vi "Example--SMO.Example.vi"() -> ()   [LabVIEW 2013]
uses:
  SMO.Example/SMO.Example.lvclass
  SMO.UI.Example/SMO.UI.Example.lvclass
  SMO.Example/Typedefs/Configuration--Cluster.ctl
  SMO.UI.Example/SMO.UI.Example.lvclass/SMO.UI.Example.ctl
  SMO.UI/SMO.UI.lvclass
  SMO/SMO.lvclass
panel:
  in  "About":bool
  out "Data Changed":string
  out "error out":errorcluster
  in  "Stop":bool
  # "SMO Example Launcher"
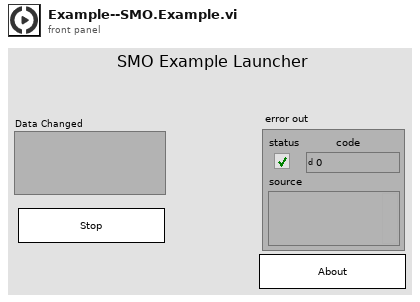
[diagram p1: front panel]
types:
  T1 = typedef "SMO.Example.lvclass/Configuration--Cluster.ctl" = cluster{"Suffix":string}
  T2 = cluster{"SMO out":refnum<class "SMO.Example.lvclass">}
  T3 = cluster{"SMO.Example Public Events":refnum<event-registration>, "SMO.UI Public Events":refnum<event-registration>}
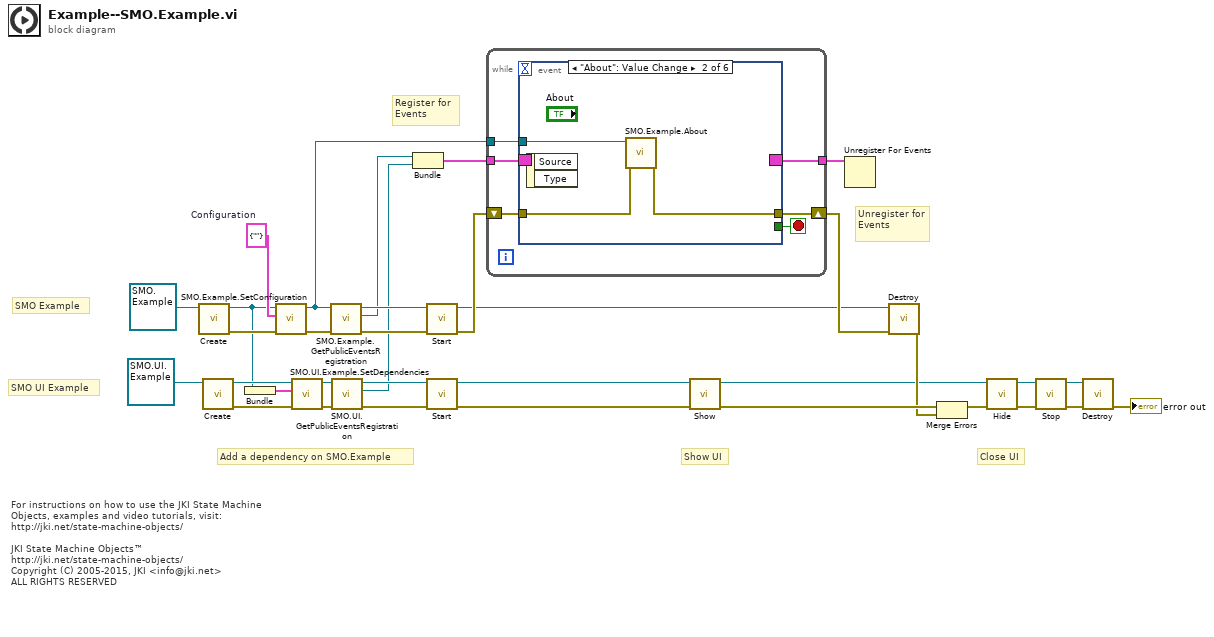
[diagram p0: block diagram]
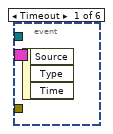
[diagram p2: hidden frame]
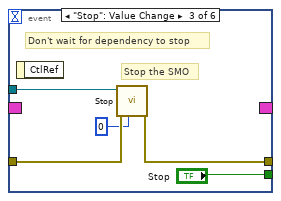
[diagram p3: hidden frame]
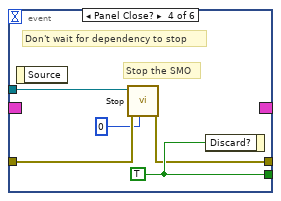
[diagram p4: hidden frame]
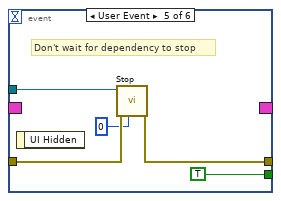
[diagram p5: hidden frame]
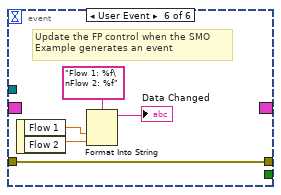
[diagram p6: hidden frame]
diagram:
  w23 = T1 {"Suffix"=""}  # Configuration
  # "Close UI"
  # "Show UI"
  # "SMO UI Example"
  # "SMO Example"
  # "For instructions on how to use the JKI State Machine Objects, examples and video tutorials, visit:\nhttp://jki.net/state-machine-objects/\n\nJKI State Machine Objects™\nhttp://jki.net/state-machine-objects/\nCopyright (C) 2005-2015, JKI <info@jki.net>\nALL RIGHTS RESERVED"
  # "Add a dependency on SMO.Example"
  # "Unregister for Events"
  # "Register for Events"
  n1 = call "Create.vi"("SMO"=refnum<class "SMO.Example.lvclass"> refnum ("SMO.Example.lvclass")) -> ("error out"=w22:errorcluster, "SMO out"=w6:refnum<class "SMO.Example.lvclass">)  [unwired: 8 in, 1 out]
  n2 = call "Create.vi"("SMO"=refnum<class "SMO.UI.Example.lvclass"> refnum ("SMO.UI.Example.lvclass")) -> ("error out"=w25:errorcluster, "SMO out"=w26:refnum<class "SMO.UI.Example.lvclass">)  [unwired: 8 in, 1 out]
  n3 = Bundle("SMO out"=w6) -> (w7:T2)  [unwired: 1 in]
  n4 = call "SMO.Example.SetConfiguration.vi"("error in (no error)"=w22, "Configuration"=w23, "SMO.Example"=w6) -> ("error out"=w18:errorcluster, "SMO.Example out"=w21:refnum<class "SMO.Example.lvclass">)  [unwired: 7 in]
  n5 = call "SMO.UI.Example.SetDependencies.vi"("error in (no error)"=w25, "Dependencies"=w7, "SMO UI.Template in"=w26) -> ("error out"=w17:errorcluster, "SMO UI.Template out"=w15:refnum<class "SMO.UI.Example.lvclass">)  [unwired: 7 in]
  n6 = call "SMO.Example.GetPublicEventsRegistration.vi"("error in (no error)"=w18, "SMO.Example"=w21) -> ("error out"=w19:errorcluster, "SMO.Example Public Events"=w12:refnum<event-registration>, "SMO.Example out"=w20:refnum<class "SMO.Example.lvclass">)  [unwired: 7 in]
  n7 = call "SMO.UI.GetPublicEventsRegistration.vi"("error in (no error)"=w17, "SMO.UI"=w15) -> ("error out"=w16:errorcluster, "SMO.UI Public Events"=w13:refnum<event-registration>, "SMO.UI out"=w14:refnum<class "SMO.UI.Example.lvclass">)  [unwired: 7 in]
  n8 = Bundle("SMO.Example Public Events"=w12, "SMO.UI Public Events"=w13) -> (w11:T3)  [unwired: 1 in]
  n9 = call "Start.vi"("error in (no error)"=w19, "SMO"=w20) -> ("error out"=w33:errorcluster, "SMO out"=w4:refnum<class "SMO.Example.lvclass">)  [unwired: 8 in]
  n10 = call "Start.vi"("error in (no error)"=w16, "SMO"=w14) -> ("error out"=w1:errorcluster, "SMO out"=w2:refnum<class "SMO.UI.Example.lvclass">)  [unwired: 8 in]
  n11 = while {
    tunnel: w21 -> [w39]
    shift-right: [w38] -> w34
    shift-left: w33 -> [w37]
    tunnel: w11 -> [w36]
    tunnel: [w35] -> w32
    stop <- w40 stop-if-true
    n12 = event shown="[1] \"About\": Value Change" {
      selector: w36 -> [_ _ _ _ _ _]
      dyn-events: [_ _ _ _ _ _] -> w35
      timeout: _ -> [_ _ _ _ _ _]
      tunnel: [_ _ "Stop" w52 TRUE ("OK") _] -> w40
      tunnel: w39 -> [_ w43 w47 w53 w58 _]
      tunnel: [_ w41 w46 w51 w55 w62] -> w38
      tunnel: w37 -> [_ w42 w45 w50 w56 w62]
      event Timeout {
        n13 = event-data() -> ()  [unwired: 1 in, 3 out]
      }
      event "About": Value Change {
        n14 = event-data() -> ()  [unwired: 1 in, 2 out]
        n15 = call "SMO.Example.About.vi"("error in (no error)"=w42, "SMO.Example"=w43) -> ("error out"=w41:errorcluster)  [unwired: 8 in, 1 out]
      }
      event "Stop": Value Change {
        # "Don't wait for dependency to stop"
        # "Stop the SMO"
        n16 = event-data() -> ()  [unwired: 1 in, 1 out]
        n17 = call "Stop.vi"("timeout in ms (-1)"=0, "error in (no error)"=w45, "SMO"=w47) -> ("error out"=w46:errorcluster)  [unwired: 7 in, 1 out]
      }
      event Panel Close? {
        w52 = TRUE ("OK")
        # "Don't wait for dependency to stop"
        # "Stop the SMO"
        n18 = event-data() -> ()  [unwired: 1 in, 1 out]
        n19 = call "Stop.vi"("timeout in ms (-1)"=0, "error in (no error)"=w50, "SMO"=w53) -> ("error out"=w51:errorcluster)  [unwired: 7 in, 1 out]
        n20 = event-data("Discard?"=w52) -> ()  [unwired: 1 in, 1 out]
      }
      event User Event {
        # "Don't wait for dependency to stop"
        n21 = event-data() -> ()  [unwired: 1 in, 1 out]
        n22 = call "Stop.vi"("timeout in ms (-1)"=0, "error in (no error)"=w56, "SMO"=w58) -> ("error out"=w55:errorcluster)  [unwired: 7 in, 1 out]
      }
      event User Event {
        # "Update the FP control when the SMO\nExample generates an event"
        n23 = event-data() -> ("Flow 1"=w60:dbl, "Flow 2"=w59:dbl)  [unwired: 1 in]
        n24 = Format Into String(format string="Flow 1: %f\nFlow 2: %f", w60, w59) -> (resulting string=→"Data Changed":string)  [unwired: 2 in, 1 out]
      }
    }
  }
  n25 = call "Show.vi"("error in (no error)"=w1, "SMO.UI"=w2) -> ("error out"=w30:errorcluster, "SMO.UI out"=w3:refnum<class "SMO.UI.Example.lvclass">)  [unwired: 8 in]
  n26 = Unregister For Events(event registration refnum=w32) -> ()  [unwired: 1 in, 1 out]
  n27 = call "Destroy.vi"("error in (no error)"=w34, "SMO"=w4) -> ("error out"=w29:errorcluster)  [unwired: 9 in]
  n28 = Merge Errors(w30, w29) -> (w28:errorcluster)
  n29 = call "Hide.vi"("error in (no error)"=w28, "SMO.UI"=w3) -> ("error out"=w5:errorcluster, "SMO.UI out"=w10:refnum<class "SMO.UI.Example.lvclass">)  [unwired: 8 in]
  n30 = call "Stop.vi"("error in (no error)"=w5, "SMO"=w10) -> ("error out"=w8:errorcluster, "SMO out"=w9:refnum<class "SMO.UI.Example.lvclass">)  [unwired: 8 in]
  n31 = call "Destroy.vi"("error in (no error)"=w8, "SMO"=w9) -> ("error out"=→"error out":errorcluster)  [unwired: 9 in]
